vi "ExampleClient.vi"() -> ()   [LabVIEW 2025]
uses:
  zeromq/Context.lvclass
  zeromq/Socket.lvclass
  libzmq-v143-mt-4_3_6/ctls/SocketOption.ctl
  libzmq-v143-mt-4_3_6/LibZMQ.lvlib
panel:
  out "data":string
  out "data":string[](array[string])
  in  "Connect":bool
  in  "ipc":bool
  in  "TCP":bool
  in  "Connection String":string
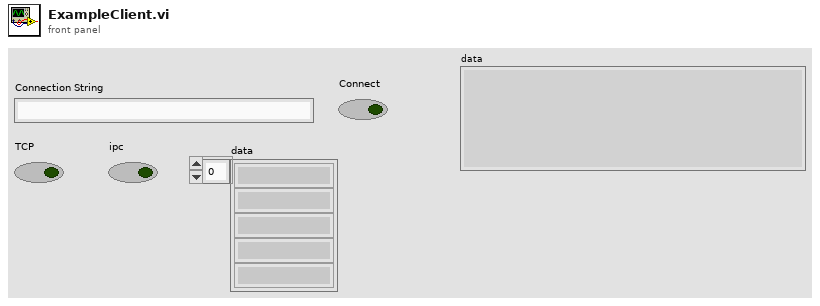
[diagram p1: front panel]
types:
  T1 = typedef "LibZMQ.lvlib/SocketOption.ctl" = enum8{"NONE", "ZMQ_HWM", "<2>", "ZMQ_SWAP", "ZMQ_AFFINITY", "ZMQ_ROUTING_ID", "ZMQ_SUBSCRIBE", "ZMQ_UNSUBSCRIBE", "ZMQ_RATE", "ZMQ_RECOVERY_IVL", "ZMQ_MCAST_LOOP", "ZMQ_SNDBUF", "ZMQ_RCVBUF", "ZMQ_RCVMORE", "ZMQ_FD", "ZMQ_EVENTS", "ZMQ_TYPE", "ZMQ_LINGER", "ZMQ_RECONNECT_IVL", "ZMQ_BACKLOG", "ZMQ_RECOVERY_IVL_MSEC", "ZMQ_RECONNECT_IVL_MAX", "ZMQ_MAXMSGSIZE", "ZMQ_SNDHWM", "ZMQ_RCVHWM", "ZMQ_MULTICAST_HOPS", "<26>", "ZMQ_RCVTIMEO", "ZMQ_SNDTIMEO", "<29>", "<30>", "ZMQ_IPV4ONLY", "ZMQ_LAST_ENDPOINT", "ZMQ_ROUTER_MANDATORY", "ZMQ_TCP_KEEPALIVE", "ZMQ_TCP_KEEPALIVE_CNT", "ZMQ_TCP_KEEPALIVE_IDLE", "ZMQ_TCP_KEEPALIVE_INTVL", "ZMQ_TCP_ACCEPT_FILTER", "ZMQ_IMMEDIATE", "ZMQ_XPUB_VERBOSE", "ZMQ_ROUTER_RAW", "ZMQ_IPV6", "ZMQ_MECHANISM", "ZMQ_PLAIN_SERVER", "ZMQ_PLAIN_USERNAME", "ZMQ_PLAIN_PASSWORD", "ZMQ_CURVE_SERVER", "ZMQ_CURVE_PUBLICKEY", "ZMQ_CURVE_SECRETKEY", "ZMQ_CURVE_SERVERKEY", "ZMQ_PROBE_ROUTER", "ZMQ_REQ_CORRELATE", "ZMQ_REQ_RELAXED", "ZMQ_CONFLATE", "ZMQ_ZAP_DOMAIN", "ZMQ_ROUTER_HANDOVER", "ZMQ_TOS", "ZMQ_IPC_FILTER_PID", "ZMQ_IPC_FILTER_UID", "ZMQ_IPC_FILTER_GID", "ZMQ_CONNECT_ROUTING_ID", "ZMQ_GSSAPI_SERVER", "ZMQ_GSSAPI_PRINCIPAL", "ZMQ_GSSAPI_SERVICE_PRINCIPAL", "ZMQ_GSSAPI_PLAINTEXT", "ZMQ_HANDSHAKE_IVL", "<67>", "ZMQ_SOCKS_PROXY", "ZMQ_XPUB_NODROP", "ZMQ_BLOCKY", "ZMQ_XPUB_MANUAL", "ZMQ_XPUB_WELCOME_MSG", "ZMQ_STREAM_NOTIFY", "ZMQ_INVERT_MATCHING", "ZMQ_HEARTBEAT_IVL", "ZMQ_HEARTBEAT_TTL", "ZMQ_HEARTBEAT_TIMEOUT", "ZMQ_XPUB_VERBOSER", "ZMQ_CONNECT_TIMEOUT", "ZMQ_TCP_MAXRT", "ZMQ_THREAD_SAFE", "<82>", "<83>", "ZMQ_MULTICAST_MAXTPDU", "ZMQ_VMCI_BUFFER_SIZE", "ZMQ_VMCI_BUFFER_MIN_SIZE", "ZMQ_VMCI_BUFFER_MAX_SIZE", "ZMQ_VMCI_CONNECT_TIMEOUT", "ZMQ_USE_FD", "ZMQ_GSSAPI_PRINCIPAL_NAMETYPE", "ZMQ_GSSAPI_SERVICE_PRINCIPAL_NAMETYPE", "ZMQ_BINDTODEVICE", "ZMQ_ZAP_ENFORCE_DOMAIN", "ZMQ_LOOPBACK_FASTPATH", "ZMQ_METADATA", "ZMQ_MULTICAST_LOOP", "ZMQ_ROUTER_NOTIFY"}
  T2 = typedef "ZeroMQ.lvlib/socket_type.ctl" = enum8{"ZMQ_PAIR", "ZMQ_PUB", "ZMQ_SUB", "ZMQ_REQ", "ZMQ_REP", "ZMQ_DEALER", "ZMQ_ROUTER", "ZMQ_PULL", "ZMQ_PUSH", "ZMQ_XPUB", "ZMQ_XSUB", "ZMQ_STREAM"}
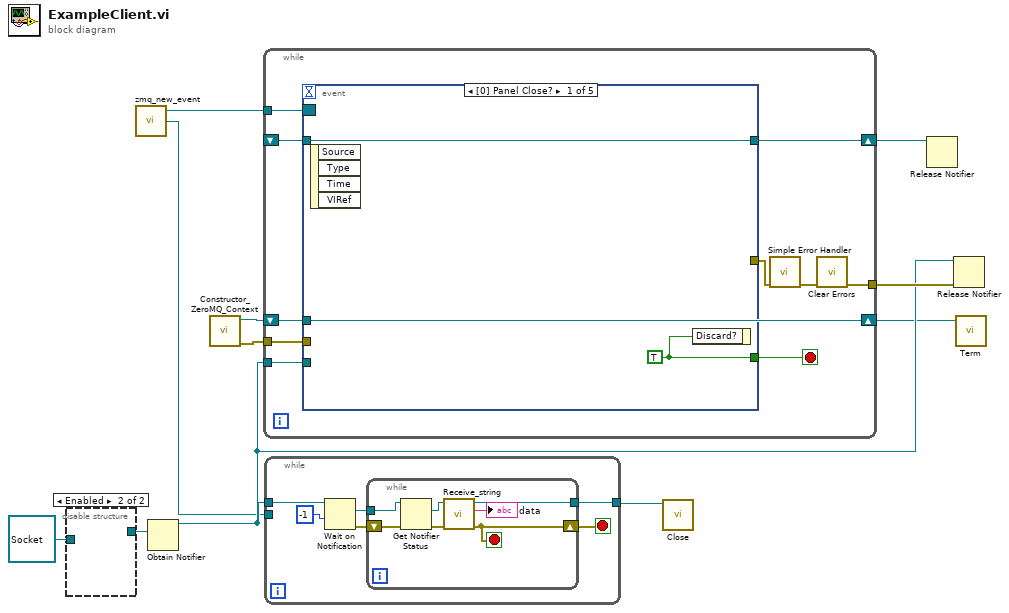
[diagram p0: block diagram]
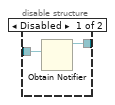
[diagram p2: hidden frame]
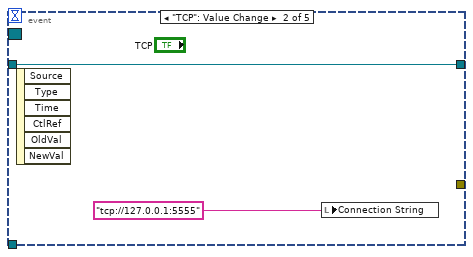
[diagram p3: hidden frame]
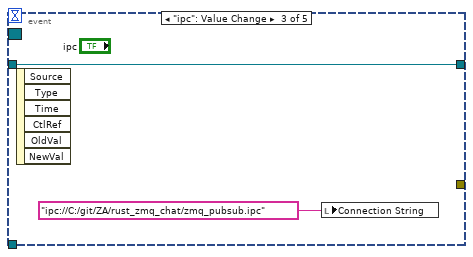
[diagram p4: hidden frame]
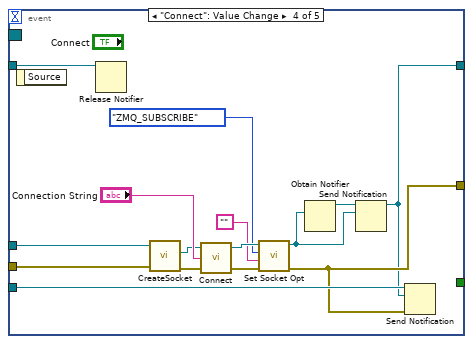
[diagram p5: hidden frame]
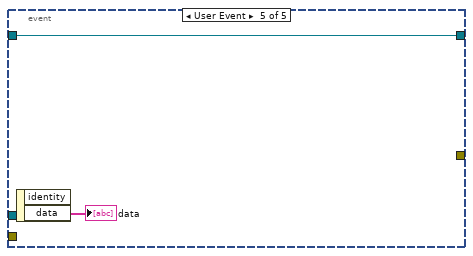
[diagram p6: hidden frame]
diagram:
  n1 = disable-structure shown="Enabled" {
    disable-tunnel: refnum<class "Socket.lvclass"> refnum ("socket out") -> [w13 _]
    disable-tunnel: [w12 _] -> w6
    frame Disabled {
      n2 = Obtain Notifier(notification data type=w13) -> (notifier out=w12:refnum<notifier>)  [unwired: 3 in, 2 out]
    }
    frame Enabled {
    }
  }
  n3 = call "zmq_new_event.vi"() -> ("user event"=w8:refnum<user-event>, "event ref out"=w11:refnum<event-registration>)  [unwired: 3 in, 1 out]
  n4 = Obtain Notifier(notification data type=w6) -> (notifier out=w9:refnum<notifier>)  [unwired: 3 in, 2 out]
  n5 = call "Constructor_ZeroMQ_Context.vi"() -> ("error out"=w4:errorcluster, "context out"=w3:refnum<class "Context.lvclass">)  [unwired: 10 in]
  n6 = while {
    tunnel: w11 -> [w21]
    tunnel: w9 -> [w20]
    tunnel: [w18] -> w10
    shift-right: [w17] -> w5
    shift-left: _ -> [w16]
    tunnel: w4 -> [w15]
    shift-right: [w14] -> w1
    shift-left: w3 -> [w14]
    stop <- w23 stop-if-true
    n7 = event shown="[0] Panel Close?" {
      selector: w21 -> [_ _ _ _ _]
      dyn-events: _ -> [_ _ _ _ _]
      timeout: _ -> [_ _ _ _ _]
      tunnel: [w25 _ _ _ _] -> w23
      tunnel: [_ _ _ w37 _] -> w22
      tunnel: w20 -> [_ _ _ w44 _]
      tunnel: [w24 w26 w28 w33 w46] -> w17
      tunnel: w16 -> [w24 w26 w28 w34 w46]
      tunnel: w15 -> [_ _ _ w31 _]
      tunnel: w14 -> [_ _ _ w30 _]
      event Panel Close? {
        w25 = TRUE
        n8 = event-data() -> ()  [unwired: 1 in, 4 out]
        n9 = event-data("Discard?"=w25) -> ()  [unwired: 1 in, 1 out]
      }
      event "TCP": Value Change {
        n10 = event-data() -> ()  [unwired: 1 in, 6 out]
        n11 = local write "Connection String"("tcp://127.0.0.1:5555") -> ()
      }
      event "ipc": Value Change {
        n12 = event-data() -> ()  [unwired: 1 in, 6 out]
        n13 = local write "Connection String"("ipc://C:/git/ZA/rust_zmq_chat/zmq_pubsub.ipc") -> ()
      }
      event "Connect": Value Change {
        n14 = event-data() -> ()  [unwired: 1 in, 1 out]
        n15 = Release Notifier(notifier=w34) -> ()  [unwired: 2 in, 3 out]
        n16 = call "CreateSocket.vi"("error in"=w31, "context in"=w30) -> ("error out"=w43:errorcluster, "socket out"=w41:refnum<class "Socket.lvclass">, "socket type"=w45:T2)  [unwired: 2 in, 1 out]
        n17 = call "Connect.vi"("error in"=w43, "endpoint"="Connection String", "socket in"=w41) -> ("error out"=w40:errorcluster, "socket out"=w39:refnum<class "Socket.lvclass">)  [unwired: 1 in]
        n18 = call "Set Socket Opt.vi"("error in"=w40, "value"="", "Socket option"=SocketOption."ZMQ_SUBSCRIBE", "socket in"=w39) -> ("error out"=w37:errorcluster, "socket out"=w32:refnum<class "Socket.lvclass">)  [unwired: 2 in]
        n19 = Obtain Notifier(notification data type=w32) -> (notifier out=w35:refnum<notifier>)  [unwired: 3 in, 2 out]
        n20 = Send Notification(notification=w32, notifier=w35) -> (notifier out=w33:refnum<notifier>)  [unwired: 1 in, 1 out]
        n21 = Send Notification(notification=w33, notifier=w44, error in (no error)=w37) -> ()  [unwired: 2 out]
      }
      event User Event {
        n22 = event-data() -> ("data"=→"data":string[])  [unwired: 1 in, 1 out]
      }
    }
    n23 = call <vilib>:"Simple Error Handler.vi"("error in (no error)"=w22) -> ("error out"=w19:errorcluster)  [unwired: 4 in, 4 out]
    n24 = call <vilib>:"Clear Errors.vi"("error in (no error)"=w19) -> ("error out"=w18:errorcluster)  [unwired: 5 in, 1 out]
  }
  n25 = while {
    tunnel: w9 -> [w53]
    tunnel: w8 -> [_]
    tunnel: [w48] -> w2
    stop <- w49 stop-if-true
    n26 = Wait on Notification(notifier=w53, timeout in ms (-1)=-1) -> (notification=w51:refnum<notifier>, error out=w50:errorcluster)  [unwired: 2 in, 2 out]
    n27 = while {
      tunnel: w51 -> [w60]
      shift-right: [w55] -> w49
      shift-left: w50 -> [w57]
      tunnel: [w54] -> w48
      stop <- w55 stop-if-true
      n28 = Get Notifier Status(notifier=w60, error in (no error)=w57) -> (current notification=w58:refnum<class "Socket.lvclass">, error out=w56:errorcluster)  [unwired: 3 out]
      n29 = call "Receive_string.vi"("error in"=w56, "socket in"=w58) -> ("error out"=w55:errorcluster, "data"=→"data":string, "socket out"=w54:refnum<class "Socket.lvclass">)  [unwired: 7 in]
    }
  }
  n30 = call "Close.vi"("socket"=w2) -> ()  [unwired: 10 in, 1 out]
  n31 = Release Notifier(notifier=w5) -> ()  [unwired: 2 in, 3 out]
  n32 = Release Notifier(notifier=w9, error in (no error)=w10) -> ()  [unwired: 1 in, 3 out]
  n33 = call "Term.vi"("context in"=w1) -> ()  [unwired: 4 in, 1 out]
